vi "MoveCursor.vi"(8 "error in (no error)":errorcluster, 10 "GameIn":refnum<class "Game.lvclass">, 11 "Highscore in":refnum<class "HighscoreDialog.lvclass">) -> (0 "error out":errorcluster, 2 "Game out":refnum<class "Game.lvclass">, 3 "Highscore out":refnum<class "HighscoreDialog.lvclass">)   [LabVIEW 2019, in "RT_Game.lvlib" / "HighscoreDialog.lvclass"]
uses:
  HighscoreDialog/HighscoreDialog.lvclass
  Game/Game.lvclass
  HighscoreDialog/HighscoreDialog.lvclass/HighscoreDialog.ctl
  Game/Game.lvclass/Game.ctl
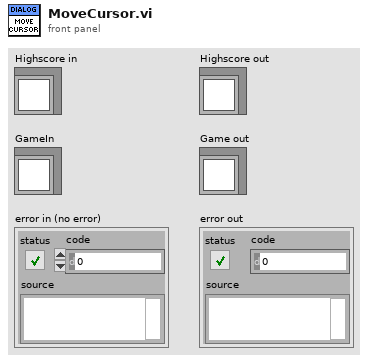
[diagram p1: front panel]
types:
  T1 = cluster{"Controls_1":cluster{"DirectionX":i8, "DirectionY":i8, "Button1":bool, "Button2":bool}, "Controls_2":cluster{"DirectionX":i8, "DirectionY":i8, "Button1":bool, "Button2":bool}, "SystemButton":bool}
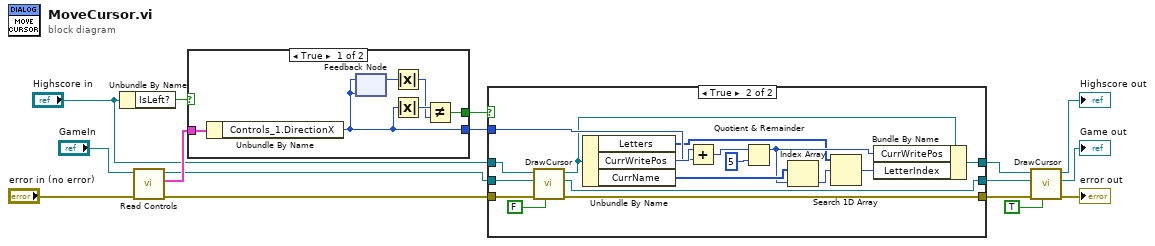
[diagram p0: block diagram]
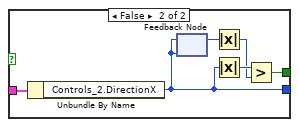
[diagram p3: hidden frame]
diagram:
  n1 = Unbundle By Name("Highscore in") -> ("IsLeft?"=w13:bool)
  n2 = call "Read Controls.vi"("error in (no error)"="error in (no error)", "Game in"="GameIn") -> ("error out"=w6:errorcluster, "Controls"=w16:T1, "Game out"=w5:refnum<class "Game.lvclass">)  [unwired: 7 in]
  n3 = case shown="True" w13 {
    tunnel: w16 -> [w22 w28]
    tunnel: [w21 w25] -> w10
    tunnel: [w19 w26] -> w11
    frame True {
      n4 = Unbundle By Name(w22) -> ("Controls_1.DirectionX"=w21:i8)
      n5 = feedback-in #1(w21) -> ()
      n6 = feedback #1(w21) -> (w20:i8)
      n7 = Absolute Value(x=w20) -> (abs(x)=w17:i8)
      n8 = Absolute Value(x=w21) -> (abs(x)=w18:i8)
      n9 = Not Equal?(x=w18, y=w17) -> (x != y?=w19:bool)
    }
    frame False {
      n10 = Unbundle By Name(w28) -> ("Controls_2.DirectionX"=w25:i8)
      n11 = feedback #2(w25) -> (w27:i8)
      n12 = feedback-in #2(w25) -> ()
      n13 = Absolute Value(x=w27) -> (abs(x)=w23:i8)
      n14 = Absolute Value(x=w25) -> (abs(x)=w24:i8)
      n15 = Greater?(x=w24, y=w23) -> (0:w26:bool)
    }
  }
  n16 = case shown="True" w11 {
    tunnel: [w31 w38] -> w2
    tunnel: "Highscore in" -> [w31 w36]
    tunnel: w10 -> [_ w46]
    tunnel: w6 -> [w30 w39]
    tunnel: w5 -> [w29 w34]
    tunnel: [w30 w37] -> w4
    tunnel: [w29 w33] -> w3
    frame False {
    }
    frame True {
      n17 = call "DrawCursor.vi"("Visible?"=FALSE, "error in (no error)"=w39, "GameIn"=w34, "Highscore in"=w36) -> ("error out"=w37:errorcluster, "GameOut"=w33:refnum<class "Game.lvclass">, "Highscore out"=w35:refnum<class "HighscoreDialog.lvclass">)  [unwired: 5 in]
      n18 = Unbundle By Name(w35) -> ("Letters"=w42:u8[], "CurrWritePos"=w48:i16, "CurrName"=w44:u8[])
      n19 = Add(x=w48, y=w46) -> (x+y=w47:i16)
      n20 = Quotient & Remainder(x=w47, y=i16 5 ("x")) -> (x-y*floor(x/y)=w43:i16)  [unwired: 1 out]
      n21 = Index Array(array=w44, index=w43) -> (element=w41:u8)
      n22 = Search 1D Array(1D array=w42, element=w41) -> (index of element=w40:i32)  [unwired: 1 in]
      n23 = Bundle By Name(cluster=w35, "CurrWritePos"=w43, "LetterIndex"=w40) -> (w38:refnum<class "HighscoreDialog.lvclass">)
    }
  }
  n24 = call "DrawCursor.vi"("Visible?"=TRUE, "error in (no error)"=w4, "GameIn"=w3, "Highscore in"=w2) -> ("error out"=→"error out":errorcluster, "GameOut"=→"Game out":refnum<class "Game.lvclass">, "Highscore out"=→"Highscore out":refnum<class "HighscoreDialog.lvclass">)  [unwired: 5 in]
